vi "invalid version.vi"() -> ()   [LabVIEW 2019]
panel:
  out "Error Out":errorcluster
  in  "TDMS File":path=path "C:/Python/projects/nitdms/tests/tdms_files/invalid version.tdms"
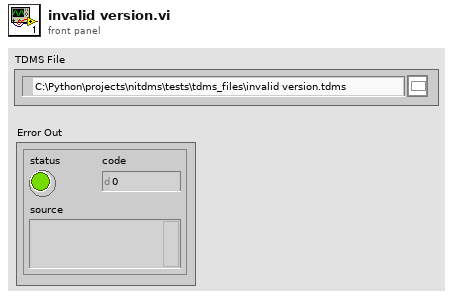
[diagram p1: front panel]
types:
  T1 = enum16{"open", "open or create", "create or replace", "create", "open (read-only)"}
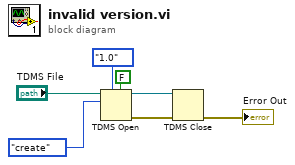
[diagram p0: block diagram]
diagram:
  n1 = TDMS Open(5:FALSE ("create index file? (T)"), 7:enum16{"1.0", "2.0"}."1.0" ("file format version (2.0)"), 10:T1."create" ("operation (0:open)"), 11:"TDMS File") -> (0:w4:errorcluster, 3:w3:refnum<k34>)  [unwired: 3 in]
  n2 = TDMS Close(8:w4, 11:w3) -> (0:→"Error Out":errorcluster)  [unwired: 1 out]
